vi "Write reference.vi"(5 "reference":refnum<vi>, 6 "error in":errorcluster, 9 "GObject in":refnum<class "Generic.lvclass">) -> (0 "error out":errorcluster, 3 "GObject out":refnum<class "Generic.lvclass">)   [LabVIEW 2014, in "Generic.lvclass"]
uses:
  Generic.lvclass
  Generic.lvclass/Generic.ctl
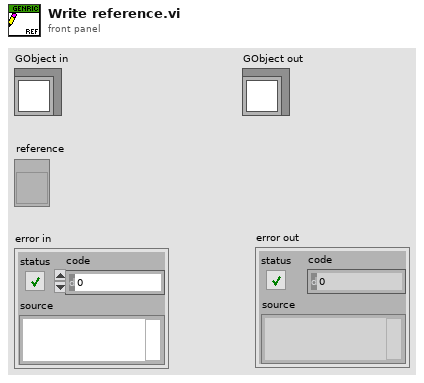
[diagram p1: front panel]
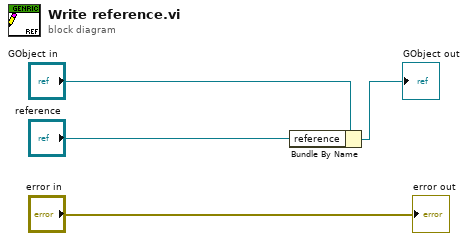
[diagram p0: block diagram]
diagram:
  n1 = Bundle By Name(cluster="GObject in", "reference"="reference") -> (→"GObject out":refnum<class "Generic.lvclass">)
  "error out" <- "error in"
